vi "dfd_2-band Lattice Coefficients Optimization Objective Function.vi"(3 "output control":T1, 4 "data":T2, 5 "X":dbl[](array[numeric])) -> (0 "error out":errorcluster, 1 "gradient":dbl[](array[numeric]), 2 "f(X)":dbl)   [LabVIEW 2017, in "NI_DigFilter_FilterBank.lvlib"]
doc: "Use this template VI as a starting point to create an objective function you want to pass to the Unconstrained Optimization VI."
uses:
  <vilib>/addons/Digital Filter Design/NI_DigFilter_FilterBank.lvlib
  <vilib>/gmath/NumericalOptimization/objective function data.ctl
  <vilib>/addons/Digital Filter Design/NI_DigFilterLicensed.lvlib
  <vilib>/gmath/NI_Gmath.lvlib
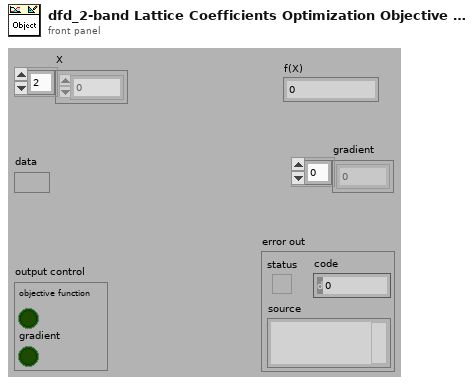
[diagram p1: front panel]
types:
  T1 = cluster{"objective function":bool, "gradient":bool}
  T2 = typedef "NI_Gmath.lvlib/objective function data.ctl" = variant
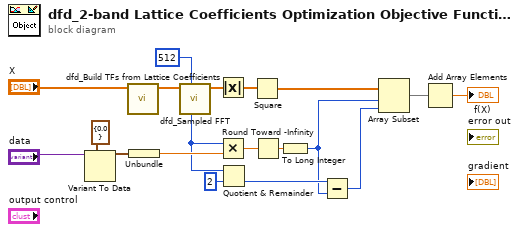
[diagram p0: block diagram]
diagram:
  w1 = 512 ("# freq bins (512)")
  n1 = Variant To Data(type=cluster{"stopband":dbl} {"stopband"=0.0} ("output cluster"), Variant="data") -> (data=w17:cluster{"stopband":dbl})  [unwired: 1 in, 1 out]
  n2 = call <vilib>:"dfd_Build TFs from Lattice Coefficients.vi"("am"="X") -> ("h0"=w14:dbl[])  [unwired: 7 in, 3 out]
  n3 = Unbundle(w17) -> ("stopband"=w12:dbl)
  n4 = call <vilib>:"dfd_Sampled FFT.vi"("# freq bins (512)"=w1, "h[n]"=w14) -> ("FFT {X}"=w6:cdb[])  [unwired: 9 in]
  n5 = Absolute Value(x=w6) -> (abs(x)=w5:dbl[])
  n6 = Multiply(x=w1, y=w12) -> (x*y=w9:dbl)
  n7 = Quotient & Remainder(x=w1, y=2) -> (floor(x/y)=w8:i32)  [unwired: 1 out]
  n8 = Square(x=w5) -> (x^2=w2:dbl[])
  n9 = Round Toward -Infinity(1:w9) -> (0:w10:dbl)
  n10 = To Long Integer(number=w10) -> (32bit integer=w4:i32)
  n11 = Subtract(x=w8, y=w4) -> (x-y=w7:i32)
  n12 = Array Subset(array=w2, index=w4, length=w7) -> (w3:dbl[])
  n13 = Add Array Elements(numeric array=w3) -> (sum=→"f(X)":dbl)
